vi "PartialClusterVI.vi"(0 "ArrayWithClusterArrays":T1(array[cluster])=[{"Numeric"=100.0, "Boolean"=TRUE, "Cluster"={"String"="1001", "Cluster"={"Numeric"=101.0, "Boolean"=TRUE, "String"="1002"}, "Boolean"=TRUE, "Numeric"=102.0}, "String"="1003", "ArrayInsideCluster"=[{"Numeric"=1.0, "Boolean"=TRUE, "Cluster"={"String"="str1A", "Cluster"={"Numeric"=2.0, "Boolean"=FALSE, "String"="str2A"}, "Boolean"=TRUE, "Numeric"=3.0}, "String"="str3A"}, {"Numeric"=10.0, "Boolean"=FALSE, "Cluster"={"String"="str10A", "Cluster"={"Numeric"=20.0, "Boolean"=TRUE, "String"="str20A"}, "Boolean"=FALSE, "Numeric"=30.0}, "String"="str30A"}]}, {"Numeric"=200.0, "Boolean"=FALSE, "Cluster"={"String"="2001", "Cluster"={"Numeric"=201.0, "Boolean"=FALSE, "String"="2002"}, "Boolean"=FALSE, "Numeric"=202.0}, "String"="2003", "ArrayInsideCluster"=[{"Numeric"=1.0, "Boolean"=TRUE, "Cluster"={"String"="str1B", "Cluster"={"Numeric"=2.0, "Boolean"=FALSE, "String"="str2B"}, "Boolean"=TRUE, "Numeric"=3.0}, "String"="str3B"}, {"Numeric"=10.0, "Boolean"=FALSE, "Cluster"={"String"="str10B", "Cluster"={"Numeric"=20.0, "Boolean"=TRUE, "String"="str20B"}, "Boolean"=FALSE, "Numeric"=30.0}, "String"="str30B"}]}], 3 "ClusterWithArray":T2={"Numeric"=0.0, "Boolean"=TRUE, "Cluster"={"String"="", "Cluster"={"Numeric"=0.0, "Boolean"=FALSE, "String"=""}, "Boolean"=FALSE, "Numeric"=0.0}, "String"="", "ArrayInsideCluster"=[{"Numeric"=1.0, "Boolean"=TRUE, "Cluster"={"String"="str1", "Cluster"={"Numeric"=2.0, "Boolean"=FALSE, "String"="str2"}, "Boolean"=TRUE, "Numeric"=3.0}, "String"="str3"}, {"Numeric"=10.0, "Boolean"=FALSE, "Cluster"={"String"="str10", "Cluster"={"Numeric"=20.0, "Boolean"=TRUE, "String"="str20"}, "Boolean"=FALSE, "Numeric"=30.0}, "String"="str30"}]}, 8 "Array":T3(array[cluster])=[{"Numeric"=1.0, "Boolean"=TRUE, "Cluster"={"String"="str1", "Cluster"={"Numeric"=2.0, "Boolean"=FALSE, "String"="str2"}, "Boolean"=TRUE, "Numeric"=3.0}, "String"="str3"}, {"Numeric"=10.0, "Boolean"=FALSE, "Cluster"={"String"="str10", "Cluster"={"Numeric"=20.0, "Boolean"=TRUE, "String"="str20"}, "Boolean"=FALSE, "Numeric"=30.0}, "String"="str30"}], 11 "Cluster":T4={"Numeric"=-1.0, "Boolean"=FALSE, "Cluster"={"String"="str-1", "Cluster"={"Numeric"=-2.0, "Boolean"=TRUE, "String"="str-2"}, "Boolean"=FALSE, "Numeric"=-3.0}, "String"="str-3"}) -> (7 "Numeric":dbl)   [LabVIEW 2012]
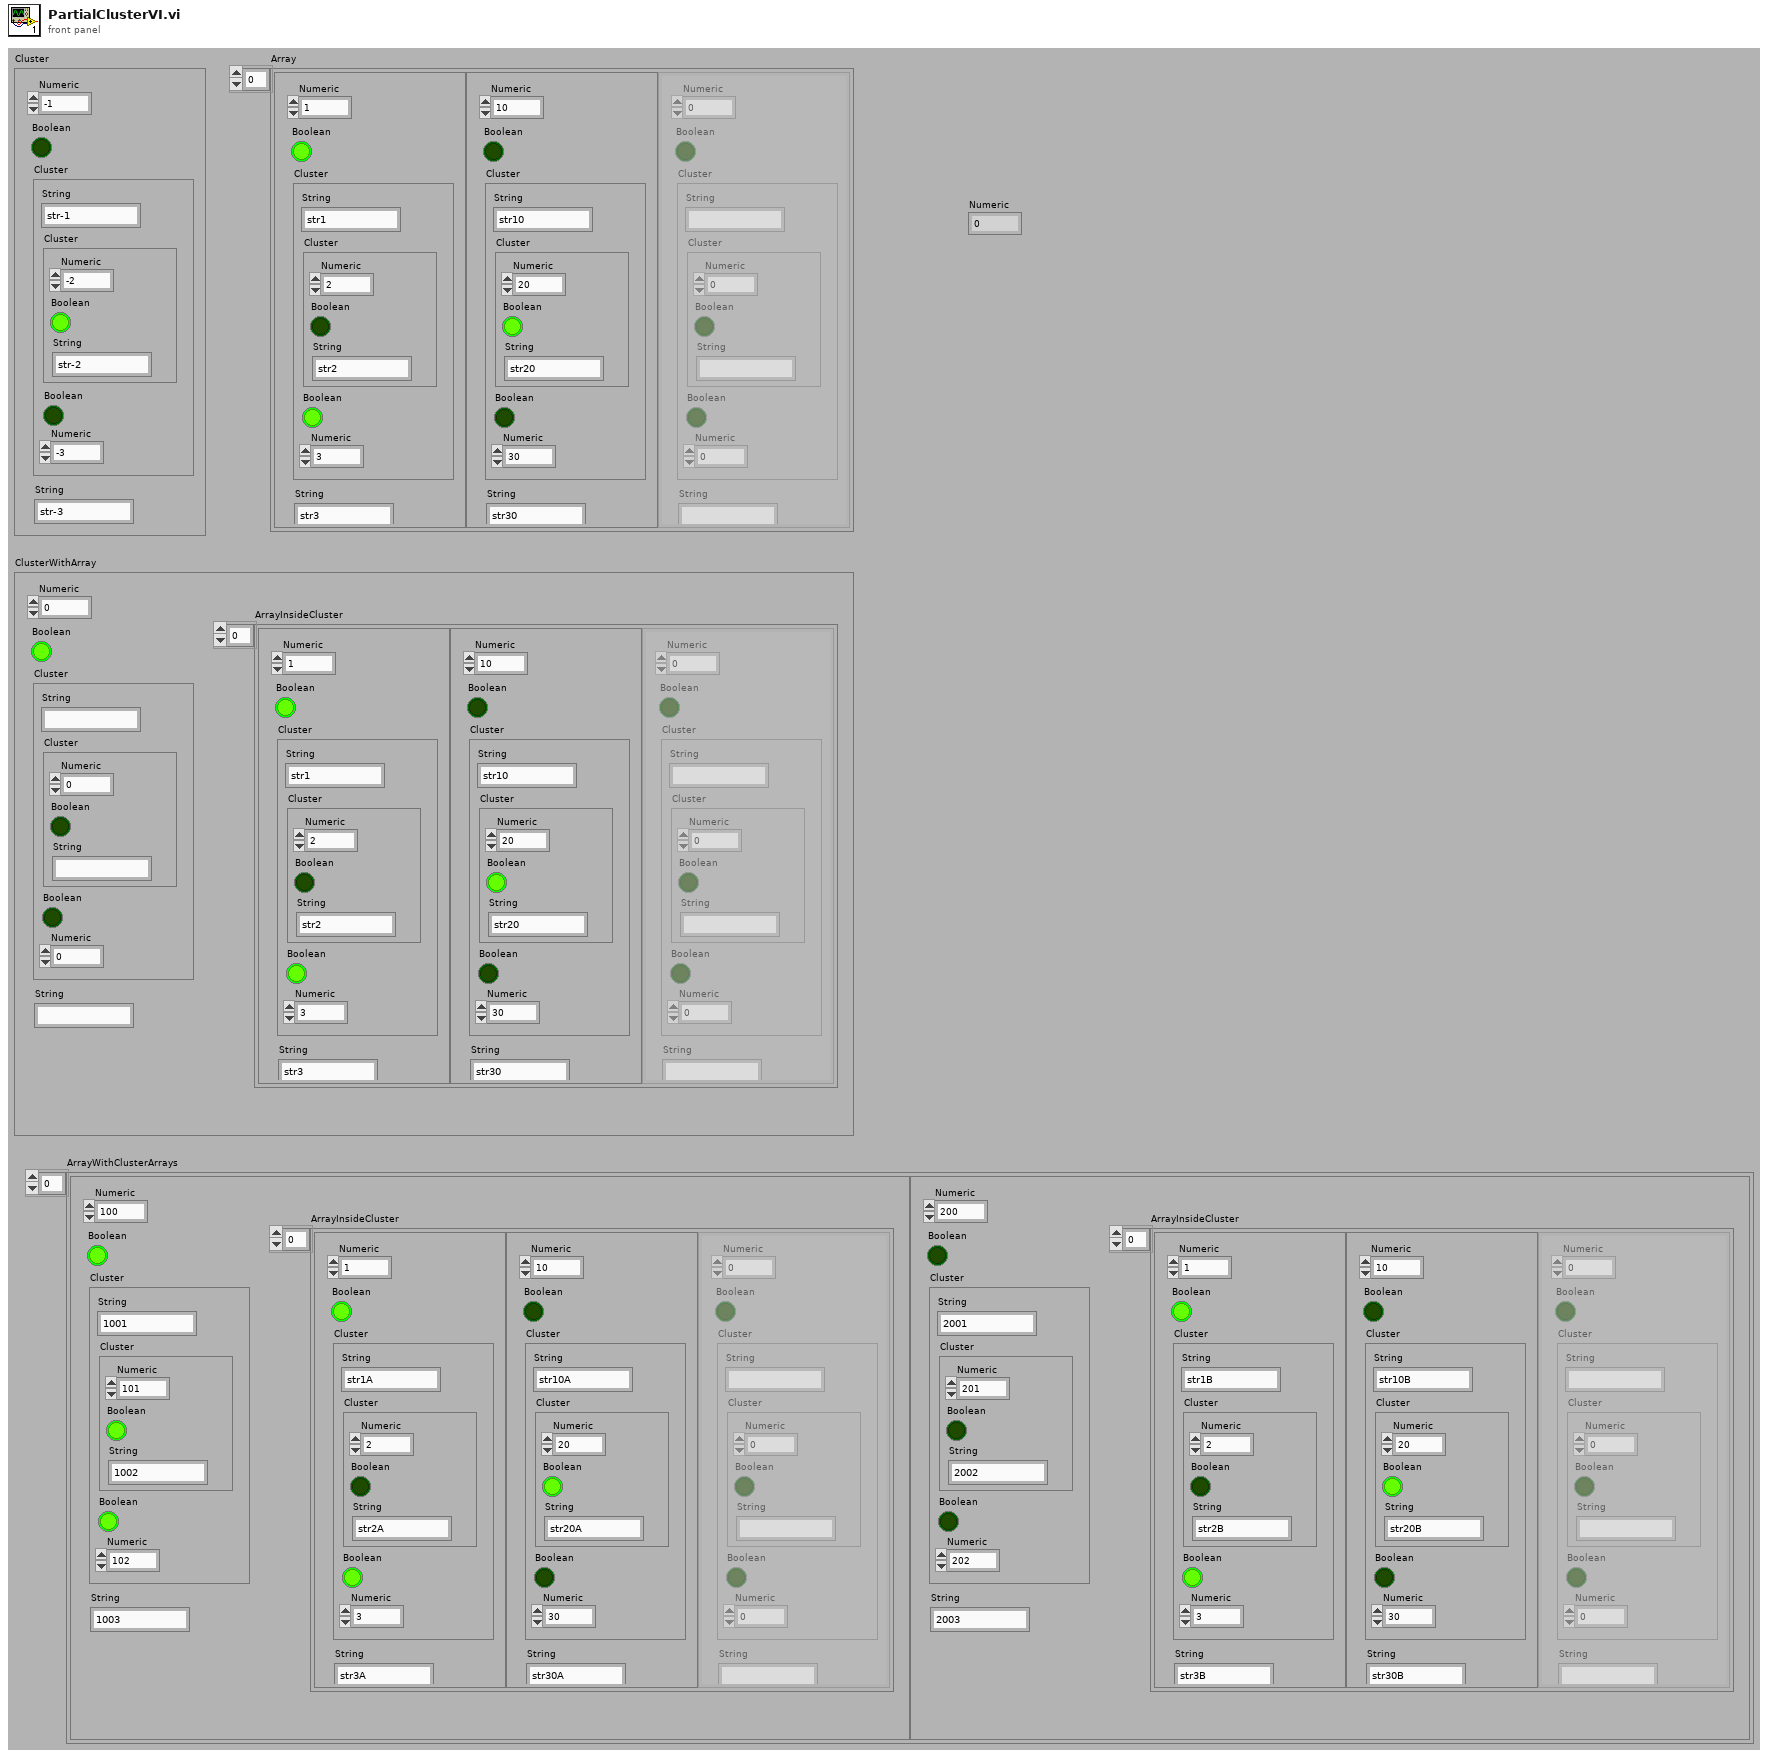
[diagram p1: front panel]
types:
  T1 = cluster{"Numeric":dbl, "Boolean":bool, "Cluster":cluster{"String":string, "Cluster":cluster{"Numeric":dbl, "Boolean":bool, "String":string}, "Boolean":bool, "Numeric":dbl}, "String":string, "ArrayInsideCluster":cluster{"Numeric":dbl, "Boolean":bool, "Cluster":cluster{"String":string, "Cluster":cluster{"Numeric":dbl, "Boolean":bool, "String":string}, "Boolean":bool, "Numeric":dbl}, "String":string}[]}[]
  T2 = cluster{"Numeric":dbl, "Boolean":bool, "Cluster":cluster{"String":string, "Cluster":cluster{"Numeric":dbl, "Boolean":bool, "String":string}, "Boolean":bool, "Numeric":dbl}, "String":string, "ArrayInsideCluster":cluster{"Numeric":dbl, "Boolean":bool, "Cluster":cluster{"String":string, "Cluster":cluster{"Numeric":dbl, "Boolean":bool, "String":string}, "Boolean":bool, "Numeric":dbl}, "String":string}[]}
  T3 = cluster{"Numeric":dbl, "Boolean":bool, "Cluster":cluster{"String":string, "Cluster":cluster{"Numeric":dbl, "Boolean":bool, "String":string}, "Boolean":bool, "Numeric":dbl}, "String":string}[]
  T4 = cluster{"Numeric":dbl, "Boolean":bool, "Cluster":cluster{"String":string, "Cluster":cluster{"Numeric":dbl, "Boolean":bool, "String":string}, "Boolean":bool, "Numeric":dbl}, "String":string}
  T5 = cluster{"String":string, "Cluster":cluster{"Numeric":dbl, "Boolean":bool, "String":string}, "Boolean":bool, "Numeric":dbl}
  T6 = cluster{"Numeric":dbl, "Boolean":bool, "String":string}
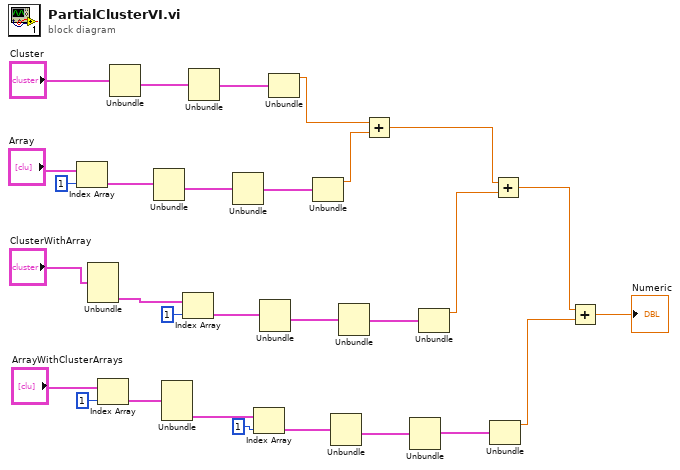
[diagram p0: block diagram]
diagram:
  n1 = Index Array(array="Array", index=1) -> (element=w21:T4)
  n2 = Unbundle("ClusterWithArray") -> ("ArrayInsideCluster"=w14:T3)  [unwired: 4 out]
  n3 = Index Array(array="ArrayWithClusterArrays", index=1) -> (element=w4:T2)
  n4 = Unbundle("Cluster") -> ("Cluster"=w28:T5)  [unwired: 3 out]
  n5 = Unbundle(w21) -> ("Cluster"=w23:T5)  [unwired: 3 out]
  n6 = Unbundle(w4) -> ("ArrayInsideCluster"=w5:T3)  [unwired: 4 out]
  n7 = Index Array(array=w14, index=1) -> (element=w15:T4)
  n8 = Unbundle(w28) -> ("Cluster"=w27:T6)  [unwired: 3 out]
  n9 = Unbundle(w23) -> ("Cluster"=w22:T6)  [unwired: 3 out]
  n10 = Index Array(array=w5, index=1) -> (element=w6:T4)
  n11 = Unbundle(w15) -> ("Cluster"=w17:T5)  [unwired: 3 out]
  n12 = Unbundle(w27) -> ("Numeric"=w26:dbl)  [unwired: 2 out]
  n13 = Unbundle(w22) -> ("Numeric"=w20:dbl)  [unwired: 2 out]
  n14 = Unbundle(w6) -> ("Cluster"=w8:T5)  [unwired: 3 out]
  n15 = Unbundle(w17) -> ("Cluster"=w16:T6)  [unwired: 3 out]
  n16 = Add(x=w26, y=w20) -> (x+y=w13:dbl)
  n17 = Unbundle(w8) -> ("Cluster"=w7:T6)  [unwired: 3 out]
  n18 = Unbundle(w16) -> ("Numeric"=w12:dbl)  [unwired: 2 out]
  n19 = Unbundle(w7) -> ("Numeric"=w2:dbl)  [unwired: 2 out]
  n20 = Add(x=w13, y=w12) -> (x+y=w3:dbl)
  n21 = Add(x=w3, y=w2) -> (x+y=→"Numeric":dbl)
